vi "extast.vi"(7 "header":string[](array[string])) -> (8 "Astrometry":T1)   [LabVIEW 2011]
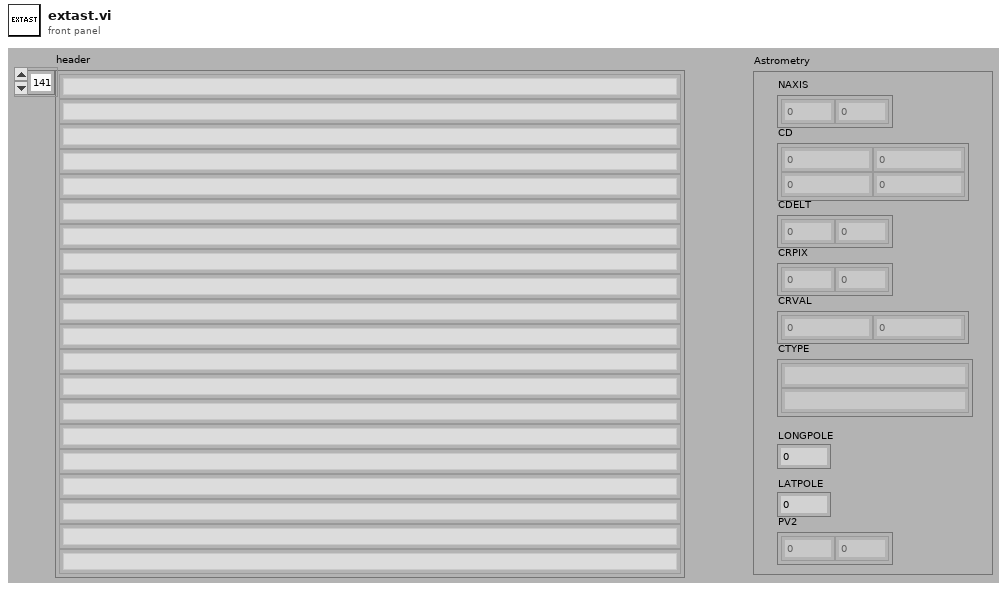
[diagram p1: front panel]
types:
  T1 = cluster{"NAXIS":dbl[], "CD":dbl[][], "CDELT":dbl[], "CRPIX":dbl[], "CTYPE":string[], "CRVAL":dbl[], "LONGPOLE":dbl, "LATPOLE":dbl, "PV2":dbl[]}
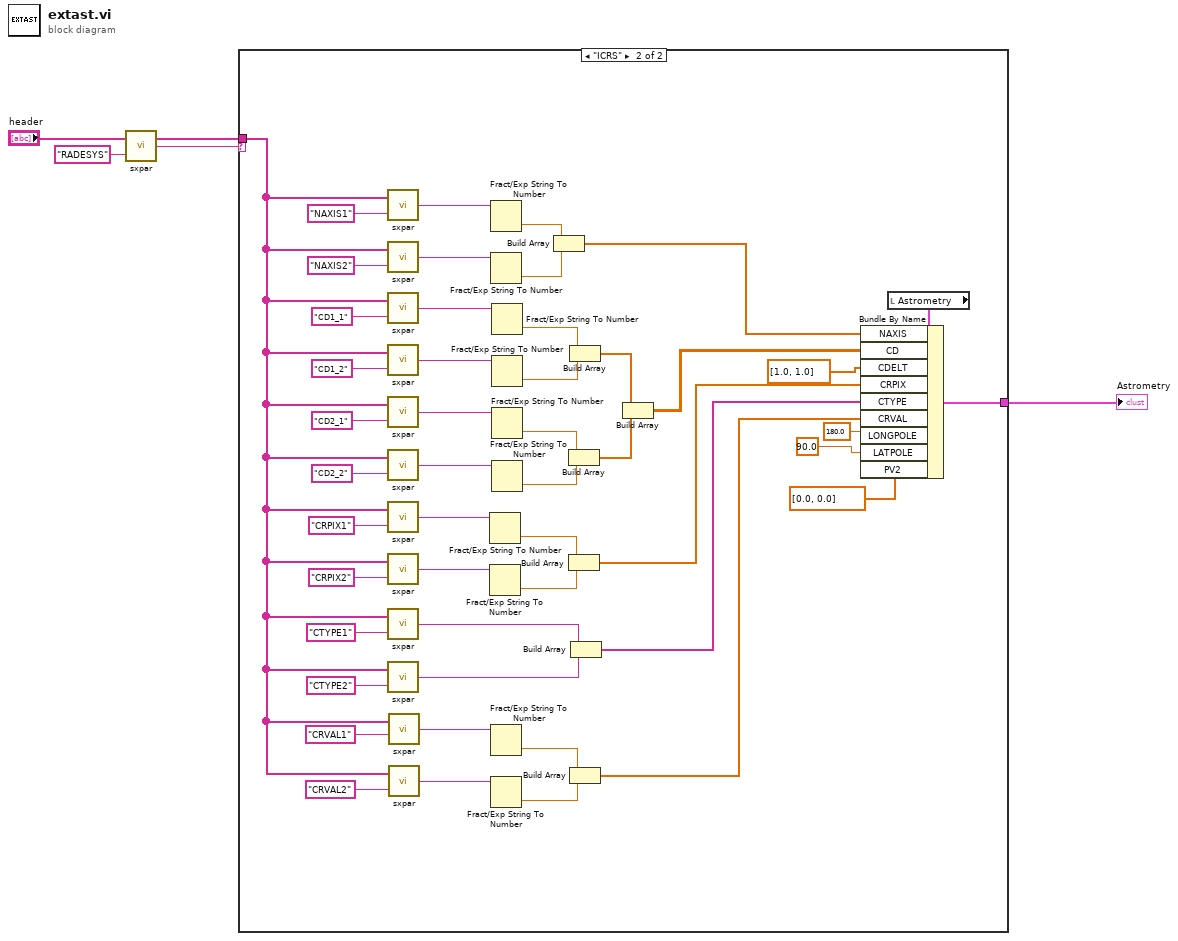
[diagram p0: block diagram]
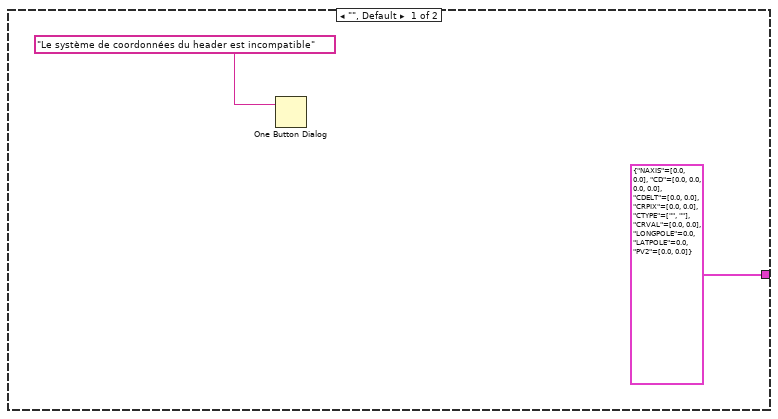
[diagram p2: hidden frame]
diagram:
  n1 = call "sxpar.vi"("Param"="RADESYS", "Array"="header") -> ("Value"=w3:string)
  n2 = case shown="\"ICRS\"" w3 {
    tunnel: "header" -> [_ w24]
    tunnel: [T1 {"NAXIS"=[0.0, 0.0], "CD"=[[0.0, 0.0], [0.0, 0.0]], "CDELT"=[0.0, 0.0], "CRPIX"=[0.0, 0.0], "CTYPE"=["", ""], "CRVAL"=[0.0, 0.0], "LONGPOLE"=0.0, "LATPOLE"=0.0, "PV2"=[0.0, 0.0]} ("Astrometry") w41] -> w1
    frame "", Default {
      n3 = One Button Dialog(message="Le système de coordonnées du header est incompatible") -> ()  [unwired: 1 in, 1 out]
    }
    frame "ICRS" {
      n4 = call "sxpar.vi"("Param"="NAXIS1", "Array"=w24) -> ("Value"=w29:string)
      n5 = call "sxpar.vi"("Param"="NAXIS2", "Array"=w24) -> ("Value"=w28:string)
      n6 = call "sxpar.vi"("Param"="CD1_1", "Array"=w24) -> ("Value"=w40:string)
      n7 = call "sxpar.vi"("Param"="CD1_2", "Array"=w24) -> ("Value"=w39:string)
      n8 = call "sxpar.vi"("Param"="CD2_1", "Array"=w24) -> ("Value"=w38:string)
      n9 = call "sxpar.vi"("Param"="CD2_2", "Array"=w24) -> ("Value"=w37:string)
      n10 = call "sxpar.vi"("Param"="CRPIX1", "Array"=w24) -> ("Value"=w21:string)
      n11 = call "sxpar.vi"("Param"="CRPIX2", "Array"=w24) -> ("Value"=w20:string)
      n12 = call "sxpar.vi"("Param"="CTYPE1", "Array"=w24) -> ("Value"=w17:string)
      n13 = call "sxpar.vi"("Param"="CTYPE2", "Array"=w24) -> ("Value"=w16:string)
      n14 = call "sxpar.vi"("Param"="CRVAL1", "Array"=w24) -> ("Value"=w14:string)
      n15 = call "sxpar.vi"("Param"="CRVAL2", "Array"=w24) -> ("Value"=w15:string)
      n16 = Fract/Exp String To Number(string=w21) -> (number=w22:dbl)  [unwired: 3 in, 1 out]
      n17 = Fract/Exp String To Number(string=w20) -> (number=w23:dbl)  [unwired: 3 in, 1 out]
      n18 = Fract/Exp String To Number(string=w29) -> (number=w27:dbl)  [unwired: 3 in, 1 out]
      n19 = Fract/Exp String To Number(string=w28) -> (number=w26:dbl)  [unwired: 3 in, 1 out]
      n20 = Fract/Exp String To Number(string=w14) -> (number=w13:dbl)  [unwired: 3 in, 1 out]
      n21 = Fract/Exp String To Number(string=w15) -> (number=w12:dbl)  [unwired: 3 in, 1 out]
      n22 = Fract/Exp String To Number(string=w40) -> (number=w34:dbl)  [unwired: 3 in, 1 out]
      n23 = Fract/Exp String To Number(string=w39) -> (number=w33:dbl)  [unwired: 3 in, 1 out]
      n24 = Fract/Exp String To Number(string=w38) -> (number=w36:dbl)  [unwired: 3 in, 1 out]
      n25 = Fract/Exp String To Number(string=w37) -> (number=w35:dbl)  [unwired: 3 in, 1 out]
      n26 = Build Array(w27, w26) -> (w25:dbl[])
      n27 = Build Array(w36, w35) -> (w32:dbl[])
      n28 = Build Array(w22, w23) -> (w19:dbl[])
      n29 = Build Array(w34, w33) -> (w31:dbl[])
      n30 = Build Array(w13, w12) -> (w11:dbl[])
      n31 = Build Array(w17, w16) -> (w18:string[])
      n32 = Build Array(w31, w32) -> (w30:dbl[][])
      n33 = local read "Astrometry"() -> (w44:T1)
      n34 = Bundle By Name(cluster=w44, "NAXIS"=w25, "CD"=w30, "CDELT"=dbl[] [1.0, 1.0], "CRPIX"=w19, "CTYPE"=w18, "CRVAL"=w11, "LONGPOLE"=180.0, "LATPOLE"=90.0, "PV2"=dbl[] [0.0, 0.0]) -> (w41:T1)
    }
  }
  "Astrometry" <- w1
